vi "数字量输入配置.vi"() -> ()   [LabVIEW 2010] (continued)
              n6448 = local write "单选_第80路"(w181) -> ()
            }
            frame 75 {
              w182 = TRUE
              w183 = FALSE ("单选_第41路")
              n6449 = local write "单选_第1路"(w182) -> ()
              n6450 = local write "单选_第2路"(w182) -> ()
              n6451 = local write "单选_第3路"(w182) -> ()
              n6452 = local write "单选_第4路"(w182) -> ()
              n6453 = local write "单选_第5路"(w182) -> ()
              n6454 = local write "单选_第6路"(w182) -> ()
              n6455 = local write "单选_第7路"(w182) -> ()
              n6456 = local write "单选_第8路"(w182) -> ()
              n6457 = local write "单选_第9路"(w182) -> ()
              n6458 = local write "单选_第10路"(w182) -> ()
              n6459 = local write "单选_第11路"(w182) -> ()
              n6460 = local write "单选_第12路"(w182) -> ()
              n6461 = local write "单选_第13路"(w182) -> ()
              n6462 = local write "单选_第14路"(w182) -> ()
              n6463 = local write "单选_第15路"(w182) -> ()
              n6464 = local write "单选_第16路"(w182) -> ()
              n6465 = local write "单选_第17路"(w182) -> ()
              n6466 = local write "单选_第18路"(w182) -> ()
              n6467 = local write "单选_第19路"(w182) -> ()
              n6468 = local write "单选_第20路"(w182) -> ()
              n6469 = local write "单选_第21路"(w182) -> ()
              n6470 = local write "单选_第22路"(w182) -> ()
              n6471 = local write "单选_第23路"(w182) -> ()
              n6472 = local write "单选_第24路"(w182) -> ()
              n6473 = local write "单选_第25路"(w182) -> ()
              n6474 = local write "单选_第26路"(w182) -> ()
              n6475 = local write "单选_第27路"(w182) -> ()
              n6476 = local write "单选_第28路"(w182) -> ()
              n6477 = local write "单选_第29路"(w182) -> ()
              n6478 = local write "单选_第30路"(w182) -> ()
              n6479 = local write "单选_第31路"(w182) -> ()
              n6480 = local write "单选_第32路"(w182) -> ()
              n6481 = local write "单选_第33路"(w182) -> ()
              n6482 = local write "单选_第34路"(w182) -> ()
              n6483 = local write "单选_第35路"(w182) -> ()
              n6484 = local write "单选_第36路"(w182) -> ()
              n6485 = local write "单选_第37路"(w182) -> ()
              n6486 = local write "单选_第38路"(w182) -> ()
              n6487 = local write "单选_第39路"(w182) -> ()
              n6488 = local write "单选_第40路"(w182) -> ()
              n6489 = local write "单选_第41路"(w182) -> ()
              n6490 = local write "单选_第42路"(w182) -> ()
              n6491 = local write "单选_第43路"(w182) -> ()
              n6492 = local write "单选_第44路"(w182) -> ()
              n6493 = local write "单选_第45路"(w182) -> ()
              n6494 = local write "单选_第46路"(w182) -> ()
              n6495 = local write "单选_第47路"(w182) -> ()
              n6496 = local write "单选_第48路"(w182) -> ()
              n6497 = local write "单选_第49路"(w182) -> ()
              n6498 = local write "单选_第50路"(w182) -> ()
              n6499 = local write "单选_第51路"(w182) -> ()
              n6500 = local write "单选_第52路"(w182) -> ()
              n6501 = local write "单选_第53路"(w182) -> ()
              n6502 = local write "单选_第54路"(w182) -> ()
              n6503 = local write "单选_第55路"(w182) -> ()
              n6504 = local write "单选_第56路"(w182) -> ()
              n6505 = local write "单选_第57路"(w182) -> ()
              n6506 = local write "单选_第58路"(w182) -> ()
              n6507 = local write "单选_第59路"(w182) -> ()
              n6508 = local write "单选_第60路"(w182) -> ()
              n6509 = local write "单选_第61路"(w182) -> ()
              n6510 = local write "单选_第62路"(w182) -> ()
              n6511 = local write "单选_第63路"(w182) -> ()
              n6512 = local write "单选_第64路"(w182) -> ()
              n6513 = local write "单选_第71路"(w182) -> ()
              n6514 = local write "单选_第79路"(w183) -> ()
              n6515 = local write "单选_第65路"(w182) -> ()
              n6516 = local write "单选_第66路"(w182) -> ()
              n6517 = local write "单选_第67路"(w182) -> ()
              n6518 = local write "单选_第68路"(w182) -> ()
              n6519 = local write "单选_第69路"(w182) -> ()
              n6520 = local write "单选_第70路"(w182) -> ()
              n6521 = local write "单选_第72路"(w182) -> ()
              n6522 = local write "单选_第73路"(w182) -> ()
              n6523 = local write "单选_第74路"(w182) -> ()
              n6524 = local write "单选_第75路"(w182) -> ()
              n6525 = local write "单选_第76路"(w183) -> ()
              n6526 = local write "单选_第77路"(w183) -> ()
              n6527 = local write "单选_第78路"(w183) -> ()
              n6528 = local write "单选_第80路"(w183) -> ()
            }
            frame 76 {
              w184 = TRUE
              w185 = FALSE ("单选_第41路")
              n6529 = local write "单选_第1路"(w184) -> ()
              n6530 = local write "单选_第2路"(w184) -> ()
              n6531 = local write "单选_第3路"(w184) -> ()
              n6532 = local write "单选_第4路"(w184) -> ()
              n6533 = local write "单选_第5路"(w184) -> ()
              n6534 = local write "单选_第6路"(w184) -> ()
              n6535 = local write "单选_第7路"(w184) -> ()
              n6536 = local write "单选_第8路"(w184) -> ()
              n6537 = local write "单选_第9路"(w184) -> ()
              n6538 = local write "单选_第10路"(w184) -> ()
              n6539 = local write "单选_第11路"(w184) -> ()
              n6540 = local write "单选_第12路"(w184) -> ()
              n6541 = local write "单选_第13路"(w184) -> ()
              n6542 = local write "单选_第14路"(w184) -> ()
              n6543 = local write "单选_第15路"(w184) -> ()
              n6544 = local write "单选_第16路"(w184) -> ()
              n6545 = local write "单选_第17路"(w184) -> ()
              n6546 = local write "单选_第18路"(w184) -> ()
              n6547 = local write "单选_第19路"(w184) -> ()
              n6548 = local write "单选_第20路"(w184) -> ()
              n6549 = local write "单选_第21路"(w184) -> ()
              n6550 = local write "单选_第22路"(w184) -> ()
              n6551 = local write "单选_第23路"(w184) -> ()
              n6552 = local write "单选_第24路"(w184) -> ()
              n6553 = local write "单选_第25路"(w184) -> ()
              n6554 = local write "单选_第26路"(w184) -> ()
              n6555 = local write "单选_第27路"(w184) -> ()
              n6556 = local write "单选_第28路"(w184) -> ()
              n6557 = local write "单选_第29路"(w184) -> ()
              n6558 = local write "单选_第30路"(w184) -> ()
              n6559 = local write "单选_第31路"(w184) -> ()
              n6560 = local write "单选_第32路"(w184) -> ()
              n6561 = local write "单选_第33路"(w184) -> ()
              n6562 = local write "单选_第34路"(w184) -> ()
              n6563 = local write "单选_第35路"(w184) -> ()
              n6564 = local write "单选_第36路"(w184) -> ()
              n6565 = local write "单选_第37路"(w184) -> ()
              n6566 = local write "单选_第38路"(w184) -> ()
              n6567 = local write "单选_第39路"(w184) -> ()
              n6568 = local write "单选_第40路"(w184) -> ()
              n6569 = local write "单选_第41路"(w184) -> ()
              n6570 = local write "单选_第42路"(w184) -> ()
              n6571 = local write "单选_第43路"(w184) -> ()
              n6572 = local write "单选_第44路"(w184) -> ()
              n6573 = local write "单选_第45路"(w184) -> ()
              n6574 = local write "单选_第46路"(w184) -> ()
              n6575 = local write "单选_第47路"(w184) -> ()
              n6576 = local write "单选_第48路"(w184) -> ()
              n6577 = local write "单选_第49路"(w184) -> ()
              n6578 = local write "单选_第50路"(w184) -> ()
              n6579 = local write "单选_第51路"(w184) -> ()
              n6580 = local write "单选_第52路"(w184) -> ()
              n6581 = local write "单选_第53路"(w184) -> ()
              n6582 = local write "单选_第54路"(w184) -> ()
              n6583 = local write "单选_第55路"(w184) -> ()
              n6584 = local write "单选_第56路"(w184) -> ()
              n6585 = local write "单选_第57路"(w184) -> ()
              n6586 = local write "单选_第58路"(w184) -> ()
              n6587 = local write "单选_第59路"(w184) -> ()
              n6588 = local write "单选_第60路"(w184) -> ()
              n6589 = local write "单选_第61路"(w184) -> ()
              n6590 = local write "单选_第62路"(w184) -> ()
              n6591 = local write "单选_第63路"(w184) -> ()
              n6592 = local write "单选_第64路"(w184) -> ()
              n6593 = local write "单选_第71路"(w184) -> ()
              n6594 = local write "单选_第79路"(w185) -> ()
              n6595 = local write "单选_第65路"(w184) -> ()
              n6596 = local write "单选_第66路"(w184) -> ()
              n6597 = local write "单选_第67路"(w184) -> ()
              n6598 = local write "单选_第68路"(w184) -> ()
              n6599 = local write "单选_第69路"(w184) -> ()
              n6600 = local write "单选_第70路"(w184) -> ()
              n6601 = local write "单选_第72路"(w184) -> ()
              n6602 = local write "单选_第73路"(w184) -> ()
              n6603 = local write "单选_第74路"(w184) -> ()
              n6604 = local write "单选_第75路"(w184) -> ()
              n6605 = local write "单选_第76路"(w184) -> ()
              n6606 = local write "单选_第77路"(w185) -> ()
              n6607 = local write "单选_第78路"(w185) -> ()
              n6608 = local write "单选_第80路"(w185) -> ()
            }
            frame 77 {
              w186 = TRUE
              w187 = FALSE ("单选_第41路")
              n6609 = local write "单选_第1路"(w186) -> ()
              n6610 = local write "单选_第2路"(w186) -> ()
              n6611 = local write "单选_第3路"(w186) -> ()
              n6612 = local write "单选_第4路"(w186) -> ()
              n6613 = local write "单选_第5路"(w186) -> ()
              n6614 = local write "单选_第6路"(w186) -> ()
              n6615 = local write "单选_第7路"(w186) -> ()
              n6616 = local write "单选_第8路"(w186) -> ()
              n6617 = local write "单选_第9路"(w186) -> ()
              n6618 = local write "单选_第10路"(w186) -> ()
              n6619 = local write "单选_第11路"(w186) -> ()
              n6620 = local write "单选_第12路"(w186) -> ()
              n6621 = local write "单选_第13路"(w186) -> ()
              n6622 = local write "单选_第14路"(w186) -> ()
              n6623 = local write "单选_第15路"(w186) -> ()
              n6624 = local write "单选_第16路"(w186) -> ()
              n6625 = local write "单选_第17路"(w186) -> ()
              n6626 = local write "单选_第18路"(w186) -> ()
              n6627 = local write "单选_第19路"(w186) -> ()
              n6628 = local write "单选_第20路"(w186) -> ()
              n6629 = local write "单选_第21路"(w186) -> ()
              n6630 = local write "单选_第22路"(w186) -> ()
              n6631 = local write "单选_第23路"(w186) -> ()
              n6632 = local write "单选_第24路"(w186) -> ()
              n6633 = local write "单选_第25路"(w186) -> ()
              n6634 = local write "单选_第26路"(w186) -> ()
              n6635 = local write "单选_第27路"(w186) -> ()
              n6636 = local write "单选_第28路"(w186) -> ()
              n6637 = local write "单选_第29路"(w186) -> ()
              n6638 = local write "单选_第30路"(w186) -> ()
              n6639 = local write "单选_第31路"(w186) -> ()
              n6640 = local write "单选_第32路"(w186) -> ()
              n6641 = local write "单选_第33路"(w186) -> ()
              n6642 = local write "单选_第34路"(w186) -> ()
              n6643 = local write "单选_第35路"(w186) -> ()
              n6644 = local write "单选_第36路"(w186) -> ()
              n6645 = local write "单选_第37路"(w186) -> ()
              n6646 = local write "单选_第38路"(w186) -> ()
              n6647 = local write "单选_第39路"(w186) -> ()
              n6648 = local write "单选_第40路"(w186) -> ()
              n6649 = local write "单选_第41路"(w186) -> ()
              n6650 = local write "单选_第42路"(w186) -> ()
              n6651 = local write "单选_第43路"(w186) -> ()
              n6652 = local write "单选_第44路"(w186) -> ()
              n6653 = local write "单选_第45路"(w186) -> ()
              n6654 = local write "单选_第46路"(w186) -> ()
              n6655 = local write "单选_第47路"(w186) -> ()
              n6656 = local write "单选_第48路"(w186) -> ()
              n6657 = local write "单选_第49路"(w186) -> ()
              n6658 = local write "单选_第50路"(w186) -> ()
              n6659 = local write "单选_第51路"(w186) -> ()
              n6660 = local write "单选_第52路"(w186) -> ()
              n6661 = local write "单选_第53路"(w186) -> ()
              n6662 = local write "单选_第54路"(w186) -> ()
              n6663 = local write "单选_第55路"(w186) -> ()
              n6664 = local write "单选_第56路"(w186) -> ()
              n6665 = local write "单选_第57路"(w186) -> ()
              n6666 = local write "单选_第58路"(w186) -> ()
              n6667 = local write "单选_第59路"(w186) -> ()
              n6668 = local write "单选_第60路"(w186) -> ()
              n6669 = local write "单选_第61路"(w186) -> ()
              n6670 = local write "单选_第62路"(w186) -> ()
              n6671 = local write "单选_第63路"(w186) -> ()
              n6672 = local write "单选_第64路"(w186) -> ()
              n6673 = local write "单选_第71路"(w186) -> ()
              n6674 = local write "单选_第79路"(w187) -> ()
              n6675 = local write "单选_第65路"(w186) -> ()
              n6676 = local write "单选_第66路"(w186) -> ()
              n6677 = local write "单选_第67路"(w186) -> ()
              n6678 = local write "单选_第68路"(w186) -> ()
              n6679 = local write "单选_第69路"(w186) -> ()
              n6680 = local write "单选_第70路"(w186) -> ()
              n6681 = local write "单选_第72路"(w186) -> ()
              n6682 = local write "单选_第73路"(w186) -> ()
              n6683 = local write "单选_第74路"(w186) -> ()
              n6684 = local write "单选_第75路"(w186) -> ()
              n6685 = local write "单选_第76路"(w186) -> ()
              n6686 = local write "单选_第77路"(w186) -> ()
              n6687 = local write "单选_第78路"(w187) -> ()
              n6688 = local write "单选_第80路"(w187) -> ()
            }
            frame 78 {
              w188 = TRUE
              w189 = FALSE ("单选_第41路")
              n6689 = local write "单选_第1路"(w188) -> ()
              n6690 = local write "单选_第2路"(w188) -> ()
              n6691 = local write "单选_第3路"(w188) -> ()
              n6692 = local write "单选_第4路"(w188) -> ()
              n6693 = local write "单选_第5路"(w188) -> ()
              n6694 = local write "单选_第6路"(w188) -> ()
              n6695 = local write "单选_第7路"(w188) -> ()
              n6696 = local write "单选_第8路"(w188) -> ()
              n6697 = local write "单选_第9路"(w188) -> ()
              n6698 = local write "单选_第10路"(w188) -> ()
              n6699 = local write "单选_第11路"(w188) -> ()
              n6700 = local write "单选_第12路"(w188) -> ()
              n6701 = local write "单选_第13路"(w188) -> ()
              n6702 = local write "单选_第14路"(w188) -> ()
              n6703 = local write "单选_第15路"(w188) -> ()
              n6704 = local write "单选_第16路"(w188) -> ()
              n6705 = local write "单选_第17路"(w188) -> ()
              n6706 = local write "单选_第18路"(w188) -> ()
              n6707 = local write "单选_第19路"(w188) -> ()
              n6708 = local write "单选_第20路"(w188) -> ()
              n6709 = local write "单选_第21路"(w188) -> ()
              n6710 = local write "单选_第22路"(w188) -> ()
              n6711 = local write "单选_第23路"(w188) -> ()
              n6712 = local write "单选_第24路"(w188) -> ()
              n6713 = local write "单选_第25路"(w188) -> ()
              n6714 = local write "单选_第26路"(w188) -> ()
              n6715 = local write "单选_第27路"(w188) -> ()
              n6716 = local write "单选_第28路"(w188) -> ()
              n6717 = local write "单选_第29路"(w188) -> ()
              n6718 = local write "单选_第30路"(w188) -> ()
              n6719 = local write "单选_第31路"(w188) -> ()
              n6720 = local write "单选_第32路"(w188) -> ()
              n6721 = local write "单选_第33路"(w188) -> ()
              n6722 = local write "单选_第34路"(w188) -> ()
              n6723 = local write "单选_第35路"(w188) -> ()
              n6724 = local write "单选_第36路"(w188) -> ()
              n6725 = local write "单选_第37路"(w188) -> ()
              n6726 = local write "单选_第38路"(w188) -> ()
              n6727 = local write "单选_第39路"(w188) -> ()
              n6728 = local write "单选_第40路"(w188) -> ()
              n6729 = local write "单选_第41路"(w188) -> ()
              n6730 = local write "单选_第42路"(w188) -> ()
              n6731 = local write "单选_第43路"(w188) -> ()
              n6732 = local write "单选_第44路"(w188) -> ()
              n6733 = local write "单选_第45路"(w188) -> ()
              n6734 = local write "单选_第46路"(w188) -> ()
              n6735 = local write "单选_第47路"(w188) -> ()
              n6736 = local write "单选_第48路"(w188) -> ()
              n6737 = local write "单选_第49路"(w188) -> ()
              n6738 = local write "单选_第50路"(w188) -> ()
              n6739 = local write "单选_第51路"(w188) -> ()
              n6740 = local write "单选_第52路"(w188) -> ()
              n6741 = local write "单选_第53路"(w188) -> ()
              n6742 = local write "单选_第54路"(w188) -> ()
              n6743 = local write "单选_第55路"(w188) -> ()
              n6744 = local write "单选_第56路"(w188) -> ()
              n6745 = local write "单选_第57路"(w188) -> ()
              n6746 = local write "单选_第58路"(w188) -> ()
              n6747 = local write "单选_第59路"(w188) -> ()
              n6748 = local write "单选_第60路"(w188) -> ()
              n6749 = local write "单选_第61路"(w188) -> ()
              n6750 = local write "单选_第62路"(w188) -> ()
              n6751 = local write "单选_第63路"(w188) -> ()
              n6752 = local write "单选_第64路"(w188) -> ()
              n6753 = local write "单选_第71路"(w188) -> ()
              n6754 = local write "单选_第79路"(w189) -> ()
              n6755 = local write "单选_第65路"(w188) -> ()
              n6756 = local write "单选_第66路"(w188) -> ()
              n6757 = local write "单选_第67路"(w188) -> ()
              n6758 = local write "单选_第68路"(w188) -> ()
              n6759 = local write "单选_第69路"(w188) -> ()
              n6760 = local write "单选_第70路"(w188) -> ()
              n6761 = local write "单选_第72路"(w188) -> ()
              n6762 = local write "单选_第73路"(w188) -> ()
              n6763 = local write "单选_第74路"(w188) -> ()
              n6764 = local write "单选_第75路"(w188) -> ()
              n6765 = local write "单选_第76路"(w188) -> ()
              n6766 = local write "单选_第77路"(w188) -> ()
              n6767 = local write "单选_第78路"(w188) -> ()
              n6768 = local write "单选_第80路"(w189) -> ()
            }
            frame 79 {
              w190 = TRUE
              n6769 = local write "单选_第1路"(w190) -> ()
              n6770 = local write "单选_第2路"(w190) -> ()
              n6771 = local write "单选_第3路"(w190) -> ()
              n6772 = local write "单选_第4路"(w190) -> ()
              n6773 = local write "单选_第5路"(w190) -> ()
              n6774 = local write "单选_第6路"(w190) -> ()
              n6775 = local write "单选_第7路"(w190) -> ()
              n6776 = local write "单选_第8路"(w190) -> ()
              n6777 = local write "单选_第9路"(w190) -> ()
              n6778 = local write "单选_第10路"(w190) -> ()
              n6779 = local write "单选_第11路"(w190) -> ()
              n6780 = local write "单选_第12路"(w190) -> ()
              n6781 = local write "单选_第13路"(w190) -> ()
              n6782 = local write "单选_第14路"(w190) -> ()
              n6783 = local write "单选_第15路"(w190) -> ()
              n6784 = local write "单选_第16路"(w190) -> ()
              n6785 = local write "单选_第17路"(w190) -> ()
              n6786 = local write "单选_第18路"(w190) -> ()
              n6787 = local write "单选_第19路"(w190) -> ()
              n6788 = local write "单选_第20路"(w190) -> ()
              n6789 = local write "单选_第21路"(w190) -> ()
              n6790 = local write "单选_第22路"(w190) -> ()
              n6791 = local write "单选_第23路"(w190) -> ()
              n6792 = local write "单选_第24路"(w190) -> ()
              n6793 = local write "单选_第25路"(w190) -> ()
              n6794 = local write "单选_第26路"(w190) -> ()
              n6795 = local write "单选_第27路"(w190) -> ()
              n6796 = local write "单选_第28路"(w190) -> ()
              n6797 = local write "单选_第29路"(w190) -> ()
              n6798 = local write "单选_第30路"(w190) -> ()
              n6799 = local write "单选_第31路"(w190) -> ()
              n6800 = local write "单选_第32路"(w190) -> ()
              n6801 = local write "单选_第33路"(w190) -> ()
              n6802 = local write "单选_第34路"(w190) -> ()
              n6803 = local write "单选_第35路"(w190) -> ()
              n6804 = local write "单选_第36路"(w190) -> ()
              n6805 = local write "单选_第37路"(w190) -> ()
              n6806 = local write "单选_第38路"(w190) -> ()
              n6807 = local write "单选_第39路"(w190) -> ()
              n6808 = local write "单选_第40路"(w190) -> ()
              n6809 = local write "单选_第41路"(w190) -> ()
              n6810 = local write "单选_第42路"(w190) -> ()
              n6811 = local write "单选_第43路"(w190) -> ()
              n6812 = local write "单选_第44路"(w190) -> ()
              n6813 = local write "单选_第45路"(w190) -> ()
              n6814 = local write "单选_第46路"(w190) -> ()
              n6815 = local write "单选_第47路"(w190) -> ()
              n6816 = local write "单选_第48路"(w190) -> ()
              n6817 = local write "单选_第49路"(w190) -> ()
              n6818 = local write "单选_第50路"(w190) -> ()
              n6819 = local write "单选_第51路"(w190) -> ()
              n6820 = local write "单选_第52路"(w190) -> ()
              n6821 = local write "单选_第53路"(w190) -> ()
              n6822 = local write "单选_第54路"(w190) -> ()
              n6823 = local write "单选_第55路"(w190) -> ()
              n6824 = local write "单选_第56路"(w190) -> ()
              n6825 = local write "单选_第57路"(w190) -> ()
              n6826 = local write "单选_第58路"(w190) -> ()
              n6827 = local write "单选_第59路"(w190) -> ()
              n6828 = local write "单选_第60路"(w190) -> ()
              n6829 = local write "单选_第61路"(w190) -> ()
              n6830 = local write "单选_第62路"(w190) -> ()
              n6831 = local write "单选_第63路"(w190) -> ()
              n6832 = local write "单选_第64路"(w190) -> ()
              n6833 = local write "单选_第71路"(w190) -> ()
              n6834 = local write "单选_第79路"(w190) -> ()
              n6835 = local write "单选_第65路"(w190) -> ()
              n6836 = local write "单选_第66路"(w190) -> ()
              n6837 = local write "单选_第67路"(w190) -> ()
              n6838 = local write "单选_第68路"(w190) -> ()
              n6839 = local write "单选_第69路"(w190) -> ()
              n6840 = local write "单选_第70路"(w190) -> ()
              n6841 = local write "单选_第72路"(w190) -> ()
              n6842 = local write "单选_第73路"(w190) -> ()
              n6843 = local write "单选_第74路"(w190) -> ()
              n6844 = local write "单选_第75路"(w190) -> ()
              n6845 = local write "单选_第76路"(w190) -> ()
              n6846 = local write "单选_第77路"(w190) -> ()
              n6847 = local write "单选_第78路"(w190) -> ()
              n6848 = local write "单选_第80路"(FALSE ("单选_第41路")) -> ()
            }
            frame 80 {
              w192 = TRUE
              n6849 = local write "单选_第1路"(w192) -> ()
              n6850 = local write "单选_第2路"(w192) -> ()
              n6851 = local write "单选_第3路"(w192) -> ()
              n6852 = local write "单选_第4路"(w192) -> ()
              n6853 = local write "单选_第5路"(w192) -> ()
              n6854 = local write "单选_第6路"(w192) -> ()
              n6855 = local write "单选_第7路"(w192) -> ()
              n6856 = local write "单选_第8路"(w192) -> ()
              n6857 = local write "单选_第9路"(w192) -> ()
              n6858 = local write "单选_第10路"(w192) -> ()
              n6859 = local write "单选_第11路"(w192) -> ()
              n6860 = local write "单选_第12路"(w192) -> ()
              n6861 = local write "单选_第13路"(w192) -> ()
              n6862 = local write "单选_第14路"(w192) -> ()
              n6863 = local write "单选_第15路"(w192) -> ()
              n6864 = local write "单选_第16路"(w192) -> ()
              n6865 = local write "单选_第17路"(w192) -> ()
              n6866 = local write "单选_第18路"(w192) -> ()
              n6867 = local write "单选_第19路"(w192) -> ()
              n6868 = local write "单选_第20路"(w192) -> ()
              n6869 = local write "单选_第21路"(w192) -> ()
              n6870 = local write "单选_第22路"(w192) -> ()
              n6871 = local write "单选_第23路"(w192) -> ()
              n6872 = local write "单选_第24路"(w192) -> ()
              n6873 = local write "单选_第25路"(w192) -> ()
              n6874 = local write "单选_第26路"(w192) -> ()
              n6875 = local write "单选_第27路"(w192) -> ()
              n6876 = local write "单选_第28路"(w192) -> ()
              n6877 = local write "单选_第29路"(w192) -> ()
              n6878 = local write "单选_第30路"(w192) -> ()
              n6879 = local write "单选_第31路"(w192) -> ()
              n6880 = local write "单选_第32路"(w192) -> ()
              n6881 = local write "单选_第33路"(w192) -> ()
              n6882 = local write "单选_第34路"(w192) -> ()
              n6883 = local write "单选_第35路"(w192) -> ()
              n6884 = local write "单选_第36路"(w192) -> ()
              n6885 = local write "单选_第37路"(w192) -> ()
              n6886 = local write "单选_第38路"(w192) -> ()
              n6887 = local write "单选_第39路"(w192) -> ()
              n6888 = local write "单选_第40路"(w192) -> ()
              n6889 = local write "单选_第41路"(w192) -> ()
              n6890 = local write "单选_第42路"(w192) -> ()
              n6891 = local write "单选_第43路"(w192) -> ()
              n6892 = local write "单选_第44路"(w192) -> ()
              n6893 = local write "单选_第45路"(w192) -> ()
              n6894 = local write "单选_第46路"(w192) -> ()
              n6895 = local write "单选_第47路"(w192) -> ()
              n6896 = local write "单选_第48路"(w192) -> ()
              n6897 = local write "单选_第49路"(w192) -> ()
              n6898 = local write "单选_第50路"(w192) -> ()
              n6899 = local write "单选_第51路"(w192) -> ()
              n6900 = local write "单选_第52路"(w192) -> ()
              n6901 = local write "单选_第53路"(w192) -> ()
              n6902 = local write "单选_第54路"(w192) -> ()
              n6903 = local write "单选_第55路"(w192) -> ()
              n6904 = local write "单选_第56路"(w192) -> ()
              n6905 = local write "单选_第57路"(w192) -> ()
              n6906 = local write "单选_第58路"(w192) -> ()
              n6907 = local write "单选_第59路"(w192) -> ()
              n6908 = local write "单选_第60路"(w192) -> ()
              n6909 = local write "单选_第61路"(w192) -> ()
              n6910 = local write "单选_第62路"(w192) -> ()
              n6911 = local write "单选_第63路"(w192) -> ()
              n6912 = local write "单选_第64路"(w192) -> ()
              n6913 = local write "单选_第71路"(w192) -> ()
              n6914 = local write "单选_第79路"(w192) -> ()
              n6915 = local write "单选_第65路"(w192) -> ()
              n6916 = local write "单选_第66路"(w192) -> ()
              n6917 = local write "单选_第67路"(w192) -> ()
              n6918 = local write "单选_第68路"(w192) -> ()
              n6919 = local write "单选_第69路"(w192) -> ()
              n6920 = local write "单选_第70路"(w192) -> ()
              n6921 = local write "单选_第72路"(w192) -> ()
              n6922 = local write "单选_第73路"(w192) -> ()
              n6923 = local write "单选_第74路"(w192) -> ()
              n6924 = local write "单选_第75路"(w192) -> ()
              n6925 = local write "单选_第76路"(w192) -> ()
              n6926 = local write "单选_第77路"(w192) -> ()
              n6927 = local write "单选_第78路"(w192) -> ()
              n6928 = local write "单选_第80路"(w192) -> ()
            }
          }
        }
      }
    }
    frame #1 {
      w194 = "DICheckStart" ("名称（未命名）")
      w197 = "DIStart" ("名称（未命名）")
      w202 = "DICheckStart" ("名称（未命名）")
      w203 = "DIStart" ("名称（未命名）")
      n6929 = Obtain Notifier(name (unnamed)=w197, notification data type=w197) -> (notifier out=w196:refnum<notifier>, error out=w195:errorcluster)  [unwired: 2 in, 1 out]
      n6930 = while {
        tunnel: w196 -> [w562]
        tunnel: w195 -> [w561]
        stop <- w563 stop-if-true
        n6931 = event shown="[15] \"btn_全选\": 值改变" {
          selector: _ -> [_ _ _ _ _ _ _ _ _ _ _ _ _ _ _ _ _ _ _]
          dyn-events: _ -> [_ _ _ _ _ _ _ _ _ _ _ _ _ _ _ _ _ _ _]
          timeout: _ -> [_ _ _ _ _ _ _ _ _ _ _ _ _ _ _ _ _ _ _]
          tunnel: [_ w564 w565 _ _ _ _ _ _ _ _ _ _ _ _ _ _ _ _] -> w563
          tunnel: w562 -> [_ _ _ _ _ _ _ _ _ _ _ _ _ w607 _ _ _ _ _]
          tunnel: w561 -> [_ _ _ _ _ _ _ _ _ _ _ _ _ w606 _ _ _ _ _]
          event Timeout {
            n6932 = event-data() -> ()  [unwired: 1 in, 2 out]
          }
          event Panel Close {
            w564 = TRUE ("关闭？")
            n6933 = event-data() -> ()  [unwired: 1 in, 3 out]
            n6934 = local write "关闭？"(w564) -> ()
          }
          event "btn_关闭": Value Change {
            w565 = TRUE
            n6935 = event-data() -> ()  [unwired: 1 in, 5 out]
            n6936 = local write "关闭？"(w565) -> ()
          }
          event "btn_全选_1": Value Change {
            n6937 = event-data() -> ("NewVal"=w567:bool)  [unwired: 1 in, 4 out]
            n6938 = case shown="假" w567 {
              tunnel: [FALSE ("单选_第41路") TRUE ("单选_第41路")] -> w566
              frame False {
              }
              frame True {
              }
            }
            n6939 = local write "单选_第1路"(w566) -> ()
            n6940 = local write "单选_第2路"(w566) -> ()
            n6941 = local write "单选_第3路"(w566) -> ()
            n6942 = local write "单选_第4路"(w566) -> ()
            n6943 = local write "单选_第5路"(w566) -> ()
            n6944 = local write "单选_第6路"(w566) -> ()
            n6945 = local write "单选_第7路"(w566) -> ()
            n6946 = local write "单选_第8路"(w566) -> ()
            n6947 = local write "单选_第9路"(w566) -> ()
            n6948 = local write "单选_第10路"(w566) -> ()
            n6949 = local write "单选_第11路"(w566) -> ()
            n6950 = local write "单选_第12路"(w566) -> ()
            n6951 = local write "单选_第13路"(w566) -> ()
            n6952 = local write "单选_第14路"(w566) -> ()
            n6953 = local write "单选_第15路"(w566) -> ()
            n6954 = local write "单选_第16路"(w566) -> ()
          }
          event "btn_全选_2": Value Change {
            n6955 = event-data() -> ("NewVal"=w571:bool)  [unwired: 1 in, 4 out]
            n6956 = case shown="假" w571 {
              tunnel: [FALSE ("单选_第41路") TRUE ("单选_第41路")] -> w570
              frame False {
              }
              frame True {
              }
            }
            n6957 = local write "单选_第17路"(w570) -> ()
            n6958 = local write "单选_第18路"(w570) -> ()
            n6959 = local write "单选_第19路"(w570) -> ()
            n6960 = local write "单选_第20路"(w570) -> ()
            n6961 = local write "单选_第21路"(w570) -> ()
            n6962 = local write "单选_第22路"(w570) -> ()
            n6963 = local write "单选_第23路"(w570) -> ()
            n6964 = local write "单选_第24路"(w570) -> ()
            n6965 = local write "单选_第25路"(w570) -> ()
            n6966 = local write "单选_第26路"(w570) -> ()
            n6967 = local write "单选_第27路"(w570) -> ()
            n6968 = local write "单选_第28路"(w570) -> ()
            n6969 = local write "单选_第29路"(w570) -> ()
            n6970 = local write "单选_第30路"(w570) -> ()
            n6971 = local write "单选_第31路"(w570) -> ()
            n6972 = local write "单选_第32路"(w570) -> ()
          }
          event "btn_全选_3": Value Change {
            n6973 = event-data() -> ("NewVal"=w575:bool)  [unwired: 1 in, 4 out]
            n6974 = case shown="假" w575 {
              tunnel: [FALSE ("单选_第41路") TRUE ("单选_第41路")] -> w574
              frame False {
              }
              frame True {
              }
            }
            n6975 = local write "单选_第33路"(w574) -> ()
            n6976 = local write "单选_第34路"(w574) -> ()
            n6977 = local write "单选_第35路"(w574) -> ()
            n6978 = local write "单选_第36路"(w574) -> ()
            n6979 = local write "单选_第37路"(w574) -> ()
            n6980 = local write "单选_第38路"(w574) -> ()
            n6981 = local write "单选_第39路"(w574) -> ()
            n6982 = local write "单选_第40路"(w574) -> ()
            n6983 = local write "单选_第41路"(w574) -> ()
            n6984 = local write "单选_第42路"(w574) -> ()
            n6985 = local write "单选_第43路"(w574) -> ()
            n6986 = local write "单选_第44路"(w574) -> ()
            n6987 = local write "单选_第45路"(w574) -> ()
            n6988 = local write "单选_第46路"(w574) -> ()
            n6989 = local write "单选_第47路"(w574) -> ()
            n6990 = local write "单选_第48路"(w574) -> ()
          }
          event "btn_全选_4": Value Change {
            n6991 = event-data() -> ("NewVal"=w579:bool)  [unwired: 1 in, 4 out]
            n6992 = case shown="假" w579 {
              tunnel: [FALSE ("单选_第41路") TRUE ("单选_第41路")] -> w578
              frame False {
              }
              frame True {
              }
            }
            n6993 = local write "单选_第49路"(w578) -> ()
            n6994 = local write "单选_第50路"(w578) -> ()
            n6995 = local write "单选_第51路"(w578) -> ()
            n6996 = local write "单选_第52路"(w578) -> ()
            n6997 = local write "单选_第53路"(w578) -> ()
            n6998 = local write "单选_第54路"(w578) -> ()
            n6999 = local write "单选_第55路"(w578) -> ()
            n7000 = local write "单选_第56路"(w578) -> ()
            n7001 = local write "单选_第57路"(w578) -> ()
            n7002 = local write "单选_第58路"(w578) -> ()
            n7003 = local write "单选_第59路"(w578) -> ()
            n7004 = local write "单选_第60路"(w578) -> ()
            n7005 = local write "单选_第61路"(w578) -> ()
            n7006 = local write "单选_第62路"(w578) -> ()
            n7007 = local write "单选_第63路"(w578) -> ()
            n7008 = local write "单选_第64路"(w578) -> ()
          }
          event "btn_全选_5": Value Change {
            n7009 = event-data() -> ("NewVal"=w583:bool)  [unwired: 1 in, 4 out]
            n7010 = case shown="假" w583 {
              tunnel: [FALSE ("单选_第41路") TRUE ("单选_第41路")] -> w582
              frame False {
              }
              frame True {
              }
            }
            n7011 = local write "单选_第71路"(w582) -> ()
            n7012 = local write "单选_第79路"(w582) -> ()
            n7013 = local write "单选_第65路"(w582) -> ()
            n7014 = local write "单选_第66路"(w582) -> ()
            n7015 = local write "单选_第67路"(w582) -> ()
            n7016 = local write "单选_第68路"(w582) -> ()
            n7017 = local write "单选_第69路"(w582) -> ()
            n7018 = local write "单选_第70路"(w582) -> ()
            n7019 = local write "单选_第72路"(w582) -> ()
            n7020 = local write "单选_第73路"(w582) -> ()
            n7021 = local write "单选_第74路"(w582) -> ()
            n7022 = local write "单选_第75路"(w582) -> ()
            n7023 = local write "单选_第76路"(w582) -> ()
            n7024 = local write "单选_第77路"(w582) -> ()
            n7025 = local write "单选_第78路"(w582) -> ()
            n7026 = local write "单选_第80路"(w582) -> ()
          }
          event "btn_置1_1": Value Change {
            n7027 = event-data() -> ("NewVal"=w587:bool)  [unwired: 1 in, 4 out]
            n7028 = case shown="假" w587 {
              tunnel: [enum16{"0", "1"}."0" ("输入值_41") enum16{"0", "1"}."1" ("输入值_41")] -> w586
              frame False {
              }
              frame True {
              }
            }
            n7029 = local write "输入值_1"(w586) -> ()
            n7030 = local write "输入值_2"(w586) -> ()
            n7031 = local write "输入值_3"(w586) -> ()
            n7032 = local write "输入值_4"(w586) -> ()
            n7033 = local write "输入值_5"(w586) -> ()
            n7034 = local write "输入值_6"(w586) -> ()
            n7035 = local write "输入值_7"(w586) -> ()
            n7036 = local write "输入值_8"(w586) -> ()
            n7037 = local write "输入值_9"(w586) -> ()
            n7038 = local write "输入值_10"(w586) -> ()
            n7039 = local write "输入值_11"(w586) -> ()
            n7040 = local write "输入值_12"(w586) -> ()
            n7041 = local write "输入值_13"(w586) -> ()
            n7042 = local write "输入值_14"(w586) -> ()
            n7043 = local write "输入值_15"(w586) -> ()
            n7044 = local write "输入值_16"(w586) -> ()
          }
          event "btn_置1_2": Value Change {
            n7045 = event-data() -> ("NewVal"=w591:bool)  [unwired: 1 in, 4 out]
            n7046 = case shown="假" w591 {
              tunnel: [enum16{"0", "1"}."0" ("输入值_41") enum16{"0", "1"}."1" ("输入值_41")] -> w590
              frame False {
              }
              frame True {
              }
            }
            n7047 = local write "输入值_17"(w590) -> ()
            n7048 = local write "输入值_18"(w590) -> ()
            n7049 = local write "输入值_19"(w590) -> ()
            n7050 = local write "输入值_20"(w590) -> ()
            n7051 = local write "输入值_21"(w590) -> ()
            n7052 = local write "输入值_22"(w590) -> ()
            n7053 = local write "输入值_23"(w590) -> ()
            n7054 = local write "输入值_24"(w590) -> ()
            n7055 = local write "输入值_25"(w590) -> ()
            n7056 = local write "输入值_26"(w590) -> ()
            n7057 = local write "输入值_27"(w590) -> ()
            n7058 = local write "输入值_28"(w590) -> ()
            n7059 = local write "输入值_29"(w590) -> ()
            n7060 = local write "输入值_30"(w590) -> ()
            n7061 = local write "输入值_31"(w590) -> ()
            n7062 = local write "输入值_32"(w590) -> ()
          }
          event "btn_置1_3": Value Change {
            n7063 = event-data() -> ("NewVal"=w595:bool)  [unwired: 1 in, 4 out]
            n7064 = case shown="假" w595 {
              tunnel: [enum16{"0", "1"}."0" ("输入值_41") enum16{"0", "1"}."1" ("输入值_41")] -> w594
              frame False {
              }
              frame True {
              }
            }
            n7065 = local write "输入值_33"(w594) -> ()
            n7066 = local write "输入值_34"(w594) -> ()
            n7067 = local write "输入值_35"(w594) -> ()
            n7068 = local write "输入值_36"(w594) -> ()
            n7069 = local write "输入值_37"(w594) -> ()
            n7070 = local write "输入值_38"(w594) -> ()
            n7071 = local write "输入值_39"(w594) -> ()
            n7072 = local write "输入值_40"(w594) -> ()
            n7073 = local write "输入值_41"(w594) -> ()
            n7074 = local write "输入值_42"(w594) -> ()
            n7075 = local write "输入值_43"(w594) -> ()
            n7076 = local write "输入值_44"(w594) -> ()
            n7077 = local write "输入值_45"(w594) -> ()
            n7078 = local write "输入值_46"(w594) -> ()
            n7079 = local write "输入值_47"(w594) -> ()
            n7080 = local write "输入值_48"(w594) -> ()
          }
          event "btn_置1_4": Value Change {
            n7081 = event-data() -> ("NewVal"=w599:bool)  [unwired: 1 in, 4 out]
            n7082 = case shown="假" w599 {
              tunnel: [enum16{"0", "1"}."0" ("输入值_41") enum16{"0", "1"}."1" ("输入值_41")] -> w598
              frame False {
              }
              frame True {
              }
            }
            n7083 = local write "输入值_49"(w598) -> ()
            n7084 = local write "输入值_50"(w598) -> ()
            n7085 = local write "输入值_51"(w598) -> ()
            n7086 = local write "输入值_52"(w598) -> ()
            n7087 = local write "输入值_53"(w598) -> ()
            n7088 = local write "输入值_54"(w598) -> ()
            n7089 = local write "输入值_55"(w598) -> ()
            n7090 = local write "输入值_56"(w598) -> ()
            n7091 = local write "输入值_57"(w598) -> ()
            n7092 = local write "输入值_58"(w598) -> ()
            n7093 = local write "输入值_59"(w598) -> ()
            n7094 = local write "输入值_60"(w598) -> ()
            n7095 = local write "输入值_61"(w598) -> ()
            n7096 = local write "输入值_62"(w598) -> ()
            n7097 = local write "输入值_63"(w598) -> ()
            n7098 = local write "输入值_64"(w598) -> ()
          }
          event "btn_置1_5": Value Change {
            n7099 = event-data() -> ("NewVal"=w603:bool)  [unwired: 1 in, 4 out]
            n7100 = case shown="假" w603 {
              tunnel: [enum16{"0", "1"}."0" ("输入值_41") enum16{"0", "1"}."1" ("输入值_41")] -> w602
              frame False {
              }
              frame True {
              }
            }
            n7101 = local write "输入值_65"(w602) -> ()
            n7102 = local write "输入值_66"(w602) -> ()
            n7103 = local write "输入值_67"(w602) -> ()
            n7104 = local write "输入值_68"(w602) -> ()
            n7105 = local write "输入值_69"(w602) -> ()
            n7106 = local write "输入值_70"(w602) -> ()
            n7107 = local write "输入值_71"(w602) -> ()
            n7108 = local write "输入值_72"(w602) -> ()
            n7109 = local write "输入值_73"(w602) -> ()
            n7110 = local write "输入值_74"(w602) -> ()
            n7111 = local write "输入值_75"(w602) -> ()
            n7112 = local write "输入值_76"(w602) -> ()
            n7113 = local write "输入值_77"(w602) -> ()
            n7114 = local write "输入值_78"(w602) -> ()
            n7115 = local write "输入值_79"(w602) -> ()
            n7116 = local write "输入值_80"(w602) -> ()
          }
          event "btn_开始试验": Value Change {
            n7117 = event-data() -> ()  [unwired: 1 in, 5 out]
            n7118 = stacked-sequence {
              tunnel: w607 -> [_ _ _ w844]
              tunnel: w606 -> [_ _ _ w843]
              frame #0 {
                w612 = 0 ("同步_A2")
                n7119 = stacked-sequence {
                  tunnel: [w636 _ _ _ _] -> w632
                  tunnel: [w635 _ _ _ _] -> w617
                  tunnel: [_ w670 _ _ _] -> w630
                  tunnel: [_ w669 _ _ _] -> w616
                  tunnel: [_ _ w704 _ _] -> w628
                  tunnel: [_ _ w703 _ _] -> w615
                  tunnel: [_ _ _ w738 _] -> w626
                  tunnel: [_ _ _ w737 _] -> w614
                  tunnel: [_ _ _ _ w772] -> w608
                  tunnel: [_ _ _ _ w771] -> w610
                  frame #0 {
                    n7120 = local read "单选_第1路"() -> (w653:bool)
                    n7121 = local read "单选_第2路"() -> (w654:bool)
                    n7122 = local read "单选_第3路"() -> (w655:bool)
                    n7123 = local read "单选_第4路"() -> (w656:bool)
                    n7124 = local read "单选_第5路"() -> (w657:bool)
                    n7125 = local read "单选_第6路"() -> (w658:bool)
                    n7126 = local read "单选_第7路"() -> (w659:bool)
                    n7127 = local read "单选_第8路"() -> (w660:bool)
                    n7128 = local read "单选_第9路"() -> (w661:bool)
                    n7129 = local read "单选_第10路"() -> (w662:bool)
                    n7130 = local read "单选_第11路"() -> (w663:bool)
                    n7131 = local read "单选_第12路"() -> (w664:bool)
                    n7132 = local read "单选_第13路"() -> (w665:bool)
                    n7133 = local read "单选_第14路"() -> (w666:bool)
                    n7134 = local read "单选_第15路"() -> (w667:bool)
                    n7135 = local read "单选_第16路"() -> (w668:bool)
                    n7136 = local read "输入值_1"() -> (w637:enum16{"0", "1"})
                    n7137 = local read "输入值_2"() -> (w638:enum16{"0", "1"})
                    n7138 = local read "输入值_3"() -> (w639:enum16{"0", "1"})
                    n7139 = local read "输入值_4"() -> (w640:enum16{"0", "1"})
                    n7140 = local read "输入值_5"() -> (w641:enum16{"0", "1"})
                    n7141 = local read "输入值_6"() -> (w642:enum16{"0", "1"})
                    n7142 = local read "输入值_7"() -> (w643:enum16{"0", "1"})
                    n7143 = local read "输入值_8"() -> (w644:enum16{"0", "1"})
                    n7144 = local read "输入值_9"() -> (w645:enum16{"0", "1"})
                    n7145 = local read "输入值_10"() -> (w646:enum16{"0", "1"})
                    n7146 = local read "输入值_11"() -> (w647:enum16{"0", "1"})
                    n7147 = local read "输入值_12"() -> (w648:enum16{"0", "1"})
                    n7148 = local read "输入值_13"() -> (w649:enum16{"0", "1"})
                    n7149 = local read "输入值_14"() -> (w650:enum16{"0", "1"})
                    n7150 = local read "输入值_15"() -> (w651:enum16{"0", "1"})
                    n7151 = local read "输入值_16"() -> (w652:enum16{"0", "1"})
                    n7152 = Build Array(w653, w654, w655, w656, w657, w658, w659, w660, w661, w662, w663, w664, w665, w666, w667, w668) -> (w636:bool[])
                    n7153 = Build Array(w637, w638, w639, w640, w641, w642, w643, w644, w645, w646, w647, w648, w649, w650, w651, w652) -> (w635:enum16{"0", "1"}[])
                  }
                  frame #1 {
                    n7154 = local read "单选_第17路"() -> (w687:bool)
                    n7155 = local read "单选_第18路"() -> (w688:bool)
                    n7156 = local read "单选_第19路"() -> (w689:bool)
                    n7157 = local read "单选_第20路"() -> (w690:bool)
                    n7158 = local read "单选_第21路"() -> (w691:bool)
                    n7159 = local read "单选_第22路"() -> (w692:bool)
                    n7160 = local read "单选_第23路"() -> (w693:bool)
                    n7161 = local read "单选_第24路"() -> (w694:bool)
                    n7162 = local read "单选_第25路"() -> (w695:bool)
                    n7163 = local read "单选_第26路"() -> (w696:bool)
                    n7164 = local read "单选_第27路"() -> (w697:bool)
                    n7165 = local read "单选_第28路"() -> (w698:bool)
                    n7166 = local read "单选_第29路"() -> (w699:bool)
                    n7167 = local read "单选_第30路"() -> (w700:bool)
                    n7168 = local read "单选_第31路"() -> (w701:bool)
                    n7169 = local read "单选_第32路"() -> (w702:bool)
                    n7170 = local read "输入值_17"() -> (w671:enum16{"0", "1"})
                    n7171 = local read "输入值_18"() -> (w672:enum16{"0", "1"})
                    n7172 = local read "输入值_19"() -> (w673:enum16{"0", "1"})
                    n7173 = local read "输入值_20"() -> (w674:enum16{"0", "1"})
                    n7174 = local read "输入值_21"() -> (w675:enum16{"0", "1"})
                    n7175 = local read "输入值_22"() -> (w676:enum16{"0", "1"})
                    n7176 = local read "输入值_23"() -> (w677:enum16{"0", "1"})
                    n7177 = local read "输入值_24"() -> (w678:enum16{"0", "1"})
                    n7178 = local read "输入值_25"() -> (w679:enum16{"0", "1"})
                    n7179 = local read "输入值_26"() -> (w680:enum16{"0", "1"})
                    n7180 = local read "输入值_27"() -> (w681:enum16{"0", "1"})
                    n7181 = local read "输入值_28"() -> (w682:enum16{"0", "1"})
                    n7182 = local read "输入值_29"() -> (w683:enum16{"0", "1"})
                    n7183 = local read "输入值_30"() -> (w684:enum16{"0", "1"})
                    n7184 = local read "输入值_31"() -> (w685:enum16{"0", "1"})
                    n7185 = local read "输入值_32"() -> (w686:enum16{"0", "1"})
                    n7186 = Build Array(w687, w688, w689, w690, w691, w692, w693, w694, w695, w696, w697, w698, w699, w700, w701, w702) -> (w670:bool[])
                    n7187 = Build Array(w671, w672, w673, w674, w675, w676, w677, w678, w679, w680, w681, w682, w683, w684, w685, w686) -> (w669:enum16{"0", "1"}[])
                  }
                  frame #2 {
                    n7188 = local read "单选_第33路"() -> (w721:bool)
                    n7189 = local read "单选_第34路"() -> (w722:bool)
                    n7190 = local read "单选_第35路"() -> (w723:bool)
                    n7191 = local read "单选_第36路"() -> (w724:bool)
                    n7192 = local read "单选_第37路"() -> (w725:bool)
                    n7193 = local read "单选_第38路"() -> (w726:bool)
                    n7194 = local read "单选_第39路"() -> (w727:bool)
                    n7195 = local read "单选_第40路"() -> (w728:bool)
                    n7196 = local read "单选_第41路"() -> (w729:bool)
                    n7197 = local read "单选_第42路"() -> (w730:bool)
                    n7198 = local read "单选_第43路"() -> (w731:bool)
                    n7199 = local read "单选_第44路"() -> (w732:bool)
                    n7200 = local read "单选_第45路"() -> (w733:bool)
                    n7201 = local read "单选_第46路"() -> (w734:bool)
                    n7202 = local read "单选_第47路"() -> (w735:bool)
                    n7203 = local read "单选_第48路"() -> (w736:bool)
                    n7204 = local read "输入值_33"() -> (w705:enum16{"0", "1"})
                    n7205 = local read "输入值_34"() -> (w706:enum16{"0", "1"})
                    n7206 = local read "输入值_35"() -> (w707:enum16{"0", "1"})
                    n7207 = local read "输入值_36"() -> (w708:enum16{"0", "1"})
                    n7208 = local read "输入值_37"() -> (w709:enum16{"0", "1"})
                    n7209 = local read "输入值_38"() -> (w710:enum16{"0", "1"})
                    n7210 = local read "输入值_39"() -> (w711:enum16{"0", "1"})
                    n7211 = local read "输入值_40"() -> (w712:enum16{"0", "1"})
                    n7212 = local read "输入值_41"() -> (w713:enum16{"0", "1"})
                    n7213 = local read "输入值_42"() -> (w714:enum16{"0", "1"})
                    n7214 = local read "输入值_43"() -> (w715:enum16{"0", "1"})
                    n7215 = local read "输入值_44"() -> (w716:enum16{"0", "1"})
                    n7216 = local read "输入值_45"() -> (w717:enum16{"0", "1"})
                    n7217 = local read "输入值_46"() -> (w718:enum16{"0", "1"})
                    n7218 = local read "输入值_47"() -> (w719:enum16{"0", "1"})
                    n7219 = local read "输入值_48"() -> (w720:enum16{"0", "1"})
                    n7220 = Build Array(w705, w706, w707, w708, w709, w710, w711, w712, w713, w714, w715, w716, w717, w718, w719, w720) -> (w703:enum16{"0", "1"}[])
                    n7221 = Build Array(w721, w722, w723, w724, w725, w726, w727, w728, w729, w730, w731, w732, w733, w734, w735, w736) -> (w704:bool[])
                  }
                  frame #3 {
                    n7222 = local read "单选_第49路"() -> (w755:bool)
                    n7223 = local read "单选_第50路"() -> (w756:bool)
                    n7224 = local read "单选_第51路"() -> (w757:bool)
                    n7225 = local read "单选_第52路"() -> (w758:bool)
                    n7226 = local read "单选_第53路"() -> (w759:bool)
                    n7227 = local read "单选_第54路"() -> (w760:bool)
                    n7228 = local read "单选_第55路"() -> (w761:bool)
                    n7229 = local read "单选_第56路"() -> (w762:bool)
                    n7230 = local read "单选_第57路"() -> (w763:bool)
                    n7231 = local read "单选_第58路"() -> (w764:bool)
                    n7232 = local read "单选_第59路"() -> (w765:bool)
                    n7233 = local read "单选_第60路"() -> (w766:bool)
                    n7234 = local read "单选_第61路"() -> (w767:bool)
                    n7235 = local read "单选_第62路"() -> (w768:bool)
                    n7236 = local read "单选_第63路"() -> (w769:bool)
                    n7237 = local read "单选_第64路"() -> (w770:bool)
                    n7238 = local read "输入值_49"() -> (w739:enum16{"0", "1"})
                    n7239 = local read "输入值_50"() -> (w740:enum16{"0", "1"})
                    n7240 = local read "输入值_51"() -> (w741:enum16{"0", "1"})
                    n7241 = local read "输入值_52"() -> (w742:enum16{"0", "1"})
                    n7242 = local read "输入值_53"() -> (w743:enum16{"0", "1"})
                    n7243 = local read "输入值_54"() -> (w744:enum16{"0", "1"})
                    n7244 = local read "输入值_55"() -> (w745:enum16{"0", "1"})
                    n7245 = local read "输入值_56"() -> (w746:enum16{"0", "1"})
                    n7246 = local read "输入值_57"() -> (w747:enum16{"0", "1"})
                    n7247 = local read "输入值_58"() -> (w748:enum16{"0", "1"})
                    n7248 = local read "输入值_59"() -> (w749:enum16{"0", "1"})
                    n7249 = local read "输入值_60"() -> (w750:enum16{"0", "1"})
                    n7250 = local read "输入值_61"() -> (w751:enum16{"0", "1"})
                    n7251 = local read "输入值_62"() -> (w752:enum16{"0", "1"})
                    n7252 = local read "输入值_63"() -> (w753:enum16{"0", "1"})
                    n7253 = local read "输入值_64"() -> (w754:enum16{"0", "1"})
                    n7254 = Build Array(w755, w756, w757, w758, w759, w760, w761, w762, w763, w764, w765, w766, w767, w768, w769, w770) -> (w738:bool[])
                    n7255 = Build Array(w739, w740, w741, w742, w743, w744, w745, w746, w747, w748, w749, w750, w751, w752, w753, w754) -> (w737:enum16{"0", "1"}[])
                  }
                  frame #4 {
                    n7256 = local read "单选_第71路"() -> (w795:bool)
                    n7257 = local read "单选_第79路"() -> (w803:bool)
                    n7258 = local read "单选_第65路"() -> (w789:bool)
                    n7259 = local read "单选_第66路"() -> (w790:bool)
                    n7260 = local read "单选_第67路"() -> (w791:bool)
                    n7261 = local read "单选_第68路"() -> (w792:bool)
                    n7262 = local read "单选_第69路"() -> (w793:bool)
                    n7263 = local read "单选_第70路"() -> (w794:bool)
                    n7264 = local read "单选_第72路"() -> (w796:bool)
                    n7265 = local read "单选_第73路"() -> (w797:bool)
                    n7266 = local read "单选_第74路"() -> (w798:bool)
                    n7267 = local read "单选_第75路"() -> (w799:bool)
                    n7268 = local read "单选_第76路"() -> (w800:bool)
                    n7269 = local read "单选_第77路"() -> (w801:bool)
                    n7270 = local read "单选_第78路"() -> (w802:bool)
                    n7271 = local read "单选_第80路"() -> (w804:bool)
                    n7272 = local read "输入值_65"() -> (w773:enum16{"0", "1"})
                    n7273 = local read "输入值_66"() -> (w774:enum16{"0", "1"})
                    n7274 = local read "输入值_67"() -> (w775:enum16{"0", "1"})
                    n7275 = local read "输入值_68"() -> (w776:enum16{"0", "1"})
                    n7276 = local read "输入值_69"() -> (w777:enum16{"0", "1"})
                    n7277 = local read "输入值_70"() -> (w778:enum16{"0", "1"})
                    n7278 = local read "输入值_71"() -> (w779:enum16{"0", "1"})
                    n7279 = local read "输入值_72"() -> (w780:enum16{"0", "1"})
                    n7280 = local read "输入值_73"() -> (w781:enum16{"0", "1"})
                    n7281 = local read "输入值_74"() -> (w782:enum16{"0", "1"})
                    n7282 = local read "输入值_75"() -> (w783:enum16{"0", "1"})
                    n7283 = local read "输入值_76"() -> (w784:enum16{"0", "1"})
                    n7284 = local read "输入值_77"() -> (w785:enum16{"0", "1"})
                    n7285 = local read "输入值_78"() -> (w786:enum16{"0", "1"})
                    n7286 = local read "输入值_79"() -> (w787:enum16{"0", "1"})
                    n7287 = local read "输入值_80"() -> (w788:enum16{"0", "1"})
                    n7288 = Build Array(w773, w774, w775, w776, w777, w778, w779, w780, w781, w782, w783, w784, w785, w786, w787, w788) -> (w771:enum16{"0", "1"}[])
                    n7289 = Build Array(w789, w790, w791, w792, w793, w794, w795, w796, w797, w798, w799, w800, w801, w802, w803, w804) -> (w772:bool[])
                  }
                }
                n7290 = local read "数组_选择?"() -> (w634:bool[][])
                n7291 = local read "数组_输入值"() -> (w618:enum16{"0", "1"}[][])
                n7292 = Replace Array Subset(array=w634, new element #1=w632, index (row) #1=0 ("索引 (行)"), new element #2=w630, index (row) #2=1 ("索引 (行)"), new element #3=w628, index (row) #3=2 ("索引 (行)"), new element #4=w626, index (row) #4=3 ("索引 (行)"), new element #5=w608, index (row) #5=4 ("索引 (行)"), new element #6=w608, index (row) #6=5 ("索引 (行)")) -> (w624:bool[][])  [unwired: 6 in]
                n7293 = Replace Array Subset(array=w618, new element #1=w617, index (row) #1=0 ("索引 (行)"), new element #2=w616, index (row) #2=1 ("索引 (行)"), new element #3=w615, index (row) #3=2 ("索引 (行)"), new element #4=w614, index (row) #4=3 ("索引 (行)"), new element #5=w610, index (row) #5=4 ("索引 (行)"), new element #6=w610, index (row) #6=5 ("索引 (行)")) -> (w613:enum16{"0", "1"}[][])  [unwired: 6 in]
                n7294 = local write "数组_选择?"(w624) -> ()
                n7295 = local write "数组_输入值"(w613) -> ()
                n7296 = local write "同步_A2"(w612) -> ()
                n7297 = local write "同步_A1"(w612) -> ()
              }
              frame #1 {
                w809 = cluster{u32, u32}[] [{9868950, 9868950}]
                n7298 = property on="light_1" class="Bool (严格)"("Colors [4]"=w809) -> ()  [unwired: 2 in, 2 out]
                n7299 = property on="light_2" class="Bool (严格)"("Colors [4]"=w809) -> ()  [unwired: 2 in, 2 out]
                n7300 = property on="light_3" class="Bool (严格)"("Colors [4]"=w809) -> ()  [unwired: 2 in, 2 out]
